vi "Controller Testing.vi"() -> ()   [LabVIEW 2014]
uses:
  <vilib>/Rock Robotics/SystemInterfaces/DIO/FPGA_DIOPWMChannel.ctl
  <vilib>/Rock Robotics/WPI/MotorControl/WPI_MotorControlOpen Talon.vi
panel:
  out "Numeric 6":dbl
  out "Numeric 5":dbl
  out "Numeric 3":dbl
  out "Numeric 2":dbl
  out "Numeric":dbl
  out "String":string
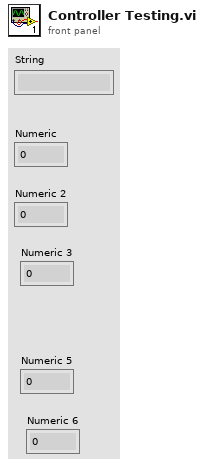
[diagram p1: front panel]
types:
  T1 = enum16{"USB 0", "USB 1", "USB 2", "USB 3", "USB 4"}
  T2 = typedef "WPI_Joystick Info.ctl" = cluster{"Device Name":string, "HID Type":T3, "XBox Type":T4, "Axes Count":i32, "Axes Types":T5[], "Button Count":i32, "POV Count":i32}
  T3 = typedef "WPI_JoystickHID Types.ctl" = enum16{"Not HID", "HID Joystick", "HID Gamepad", "HID Driving Wheel", "HID Flightstick", "HID First Person"}
  T4 = typedef "WPI_JoystickXBox Types.ctl" = enum16{"Not XBox", "XBox Unknown", "XBox Gamepad", "XBox Wheel", "XBox Arcade Stick", "XBox Flight Stick", "XBox Dance Pad", "XBox Guitar", "XBox Drum Kit", "XBox Arcade Pad"}
  T5 = typedef "WPI_JoystickAxis Types.ctl" = enum16{"X Axis", "Y Axis", "Z Axis", "RxAxis", "RyAxis", "RzAxis", "Slider", "POV", "None", "L X Axis", "L Y Axis", "L Trigger", "R Trigger", "R X Axis", "R Y Axis"}
  T6 = typedef "FPGA_DIOPWMChannel.ctl" = enum8{"PWM 0", "PWM 1", "PWM 2", "PWM 3", "PWM 4", "PWM 5", "PWM 6", "PWM 7", "PWM 8", "PWM 9", "PWM MXP 0", "PWM MXP 1", "PWM MXP 2", "PWM MXP 3", "PWM MXP 4", "PWM MXP 5", "PWM MXP 6", "PWM MXP 7", "PWM MXP 8", "PWM MXP 9", "Invalid"}
  T7 = typedef "WPI_MotorControlDeviceRef.ctl" = cluster{"DeviceStatus":errorcluster, "Type":T8, "PWM":cluster{"Controller":T9, "PWM Channel":T6, "DeadBand":T10}, "CAN":cluster{"Device Number":u8, "Control Mode":T11, "Semaphore":T12, "Max Vout":dbl, "TalonSRX Control Mode":T13}, "Invert":bool, "TransformRef":T14, "InvTransformRef":T14}
  T8 = typedef "WPI_MotorControlType.ctl" = enum16{"PWM", "CAN", "CANTalonSRX"}
  T9 = typedef "FPGA_TypedefDigitalModule.ctl" = enum16{"Controller 1"}
  T10 = typedef "WPI_PWMDeadband.ctl" = cluster{"Name":string, "maxPositivePwm":i32, "minPositivePwm":i32, "centerPwm":i32, "maxNegativePwm":i32, "minNegativePwm":i32, "angularRange":u16}
  T11 = typedef "WPI_CANJaguar_ControlMode.ctl" = enum8{"Percent VBus", "Current", "Speed", "Position", "Voltage"}
  T12 = typedef "Semaphore RefNum" = refnum<k1>
  T13 = typedef "WPI_CANTalonSRX_APIControlMode.ctl" = enum8{"Percent VBus", "Speed", "Position", "Slave", "Unchanged / Invalid"}
  T14 = typedef "WPI_PWMTransform_ConPane.ctl" = refnum<vi>
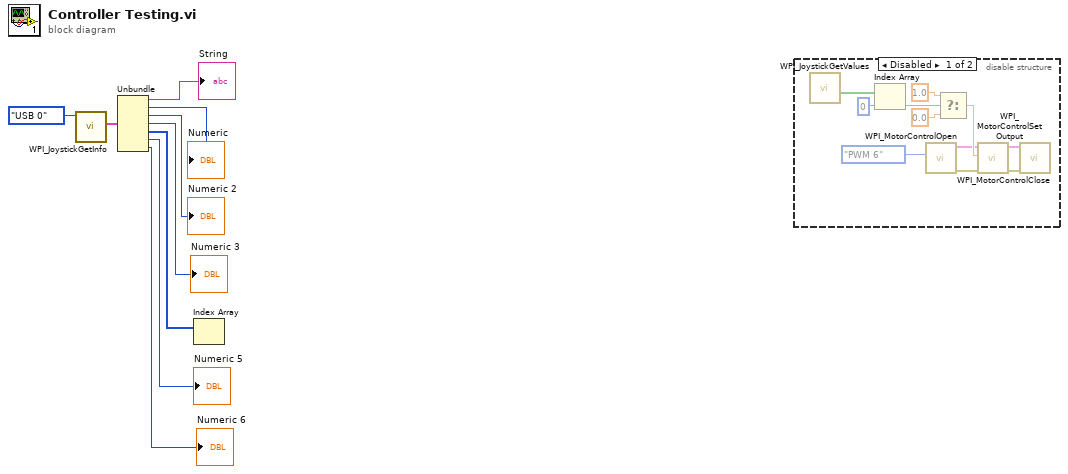
[diagram p0: block diagram]
diagram:
  n1 = call <vilib>:"WPI_JoystickGetInfo.vi"("JoystickDevice"=T1."USB 0") -> ("Joystick Info"=w8:T2)  [unwired: 9 in, 1 out]
  n2 = Unbundle(w8) -> ("Device Name"=→"String":string, "HID Type"=→"Numeric":T3, "XBox Type"=→"Numeric 2":T4, "Axes Count"=→"Numeric 3":i32, "Axes Types"=w1:T5[], "Button Count"=→"Numeric 5":i32, "POV Count"=→"Numeric 6":i32)
  n3 = Index Array(array=w1) -> ()  [unwired: 1 in, 1 out]
  n4 = disable-structure shown="Disabled" {
    frame Disabled {
      n5 = call <vilib>:"WPI_JoystickGetValues.vi"() -> ("Buttons"=w20:bool[])  [unwired: 7 in, 4 out]
      n6 = Index Array(array=w20, index=0) -> (element=w18:bool)
      n7 = call-poly <vilib>:"WPI_MotorControlOpen.vi"("PWM Channel"=FPGA_DIOPWMChannel."PWM 6") -> ("error out"=w13:errorcluster, "MotorControlDeviceRef"=w14:T7)  [unwired: 9 in]
      n8 = Select(t=1.0, s=w18, f=0.0) -> (s? t:f=w15:dbl)
      n9 = call <vilib>:"WPI_MotorControlSetOutput.vi"("error in (no error)"=w13, "Output"=w15, "MotorControlDevRef"=w14) -> ("error out"=w10:errorcluster, "MotorControlDevRef"=w11:T7)  [unwired: 6 in, 1 out]
      n10 = call <vilib>:"WPI_MotorControlClose.vi"("error in (no error)"=w10, "MotorControlDevRef"=w11) -> ()  [unwired: 9 in, 1 out]
    }
    frame Enabled {
    }
  }
